vi "get wavemakerfile.vi"(6 "warning":bool=TRUE, 7 "file path":path) -> (0 "discontinuities":bool, 3 "waveform":sgl[](array[numeric]) format="%.2f", 5 "new file path":path)   [LabVIEW 2010]
uses:
  <vilib>/Utility/file.llb/Read From Spreadsheet File (DBL).vi
  <vilib>/Analysis/NI_AALPro.lvlib
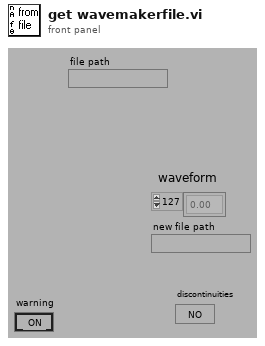
[diagram p1: front panel]
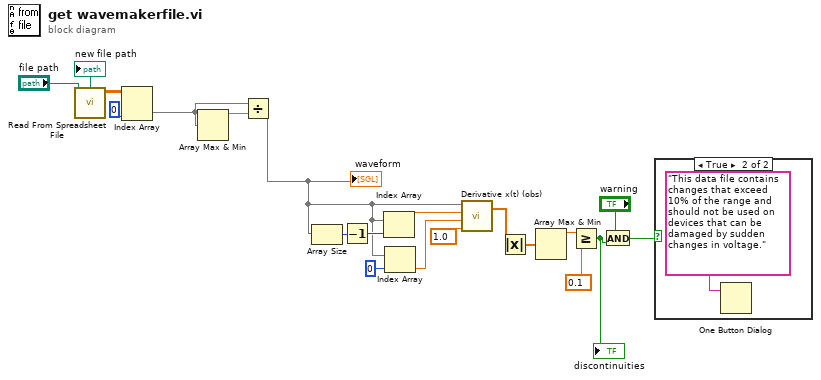
[diagram p0: block diagram]
diagram:
  n1 = call-poly <vilib>:"Read From Spreadsheet File.vi"("file path (dialog if empty)"="file path") -> ("all rows"=w20:dbl[][], "new file path (Not A Path if cancelled)"=→"new file path":path)  [unwired: 6 in, 3 out]
  n2 = Index Array(array=w20, index (col)=0) -> (element=w15:dbl[])  [unwired: 1 in]
  n3 = Array Max & Min(array=w15) -> (max value=w16:dbl)  [unwired: 3 out]
  n4 = Divide(x=w15, y=w16) -> (x/y=w1:dbl[])
  "waveform" <- w1
  n5 = Array Size(array=w1) -> (size(s)=w13:i32)
  n6 = Decrement(x=w13) -> (x-1=w12:i32)
  n7 = Index Array(array=w1, index=w12) -> (element=w11:dbl)
  n8 = Index Array(array=w1, index=0) -> (element=w10:dbl)
  n9 = call <vilib>:"Derivative x(t) (obs).vi"("dt"=1.0, "final condition"=w10, "initial condition"=w11, "X"=w1) -> ("dX/dt"=w8:dbl[])  [unwired: 1 out]
  n10 = Absolute Value(x=w8) -> (abs(x)=w7:dbl[])
  n11 = Array Max & Min(array=w7) -> (max value=w6:dbl)  [unwired: 3 out]
  n12 = Greater Or Equal?(x=w6, y=0.1) -> (x >= y?=w2:bool)
  "discontinuities" <- w2
  n13 = And(x="warning", y=w2) -> (x .and. y?=w4:bool)
  n14 = case shown="True" w4 {
    frame False {
    }
    frame True {
      n15 = One Button Dialog(message="This data file contains changes that exceed 10% of the range and should not be used on devices that can be damaged by sudden changes in voltage.") -> ()  [unwired: 1 in, 1 out]
    }
  }
